vi "SSL Detection Balls Delete Invalids.vi"(5 "Now":timestamp, 7 "Life Time":dbl=1.0, 11 "Balls in":refnum<class "Ball.lvclass">[](array[class])) -> (3 "Balls out":refnum<class "Ball.lvclass">[](array[class]))   [LabVIEW 2018]
uses:
  Ball_class/Ball.lvclass
  Ball_class/Ball.lvclass/Ball.ctl
  Ball_class/Read Valid.vi
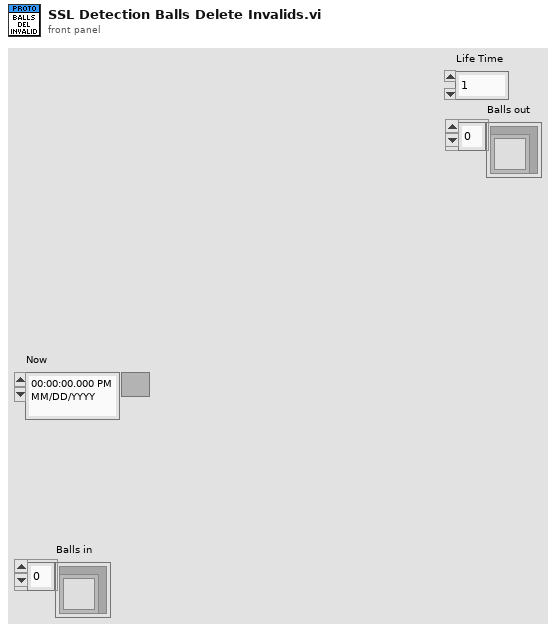
[diagram p1: front panel]
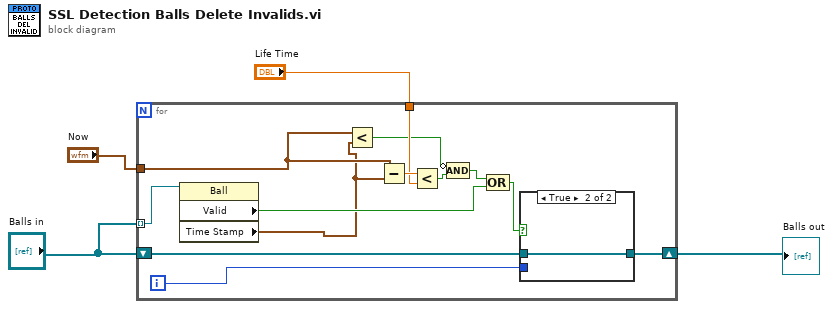
[diagram p0: block diagram]
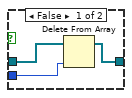
[diagram p2: hidden frame]
diagram:
  n1 = for {
    tunnel: "Balls in" -> [w7] mode=indexing
    shift-right: [w15] -> w4
    shift-left: "Balls in" -> [w17]
    tunnel: "Now" -> [w11]
    tunnel: "Life Time" -> [w13]
    i -> [w16]
    n2 = property class="Ball"(reference=w7) -> ("Valid"=w6:bool, "Time Stamp"=w5:timestamp)  [unwired: 1 in, 2 out]
    n3 = Less?(x=w11, y=w5) -> (x < y?=w9:bool)
    n4 = Subtract(x=w11, y=w5) -> (x-y=w14:dbl)
    n5 = Less?(x=w14, y=w13) -> (x < y?=w10:bool)
    n6 = Compound Arithmetic op=AND(invert w9, w10) -> (w8:bool)
    n7 = Compound Arithmetic op=OR(w8, w6) -> (w12:bool)
    n8 = case shown="True" w12 {
      tunnel: w17 -> [w20 w21]
      tunnel: w16 -> [w19 _]
      tunnel: [w18 w21] -> w15
      frame False {
        n9 = Delete From Array(array=w20, index=w19) -> (array with subset deleted=w18:refnum<class "Ball.lvclass">[])  [unwired: 1 in, 1 out]
      }
      frame True {
      }
    }
  }
  "Balls out" <- w4
